vi "Part A.vi"() -> ()   [LabVIEW 2020]
uses:
  <vilib>/MakerHub/LINX/Public/Peripherals/Digital/Digital Write N Chans.vi
  <vilib>/MakerHub/LINX/Private/Local IO/LinxDigitalWrite.vi
  <vilib>/MakerHub/LINX/Public/Utilities/Check Channel.vi
  <vilib>/MakerHub/LINX/Public/Utilities/Open Serial.vi
  <vilib>/MakerHub/LINX/Private/Utilties/Generate Error.vi
  <vilib>/MakerHub/LINX/LMH-LINX.lvlib
panel:
  in  "?":bool
  in  "Serial Port":refnum<visa-resource-name>="N/A"
  in  "Slide":dbl(slide) scale=0.0..4.0
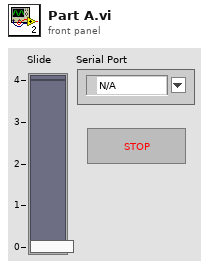
[diagram p1: front panel]
types:
  T1 = typedef "LMH-LINX.lvlib/LINX Ref.ctl" = cluster{"IO":T2, "Interface":T3, "LINX Device Config":T4}
  T2 = typedef "LMH-LINX.lvlib/Platform.ctl" = enum16{"Remote", "Local"}
  T3 = typedef "LMH-LINX.lvlib/Interface.ctl" = enum16{"Serial", "TCP"}
  T4 = typedef "LMH-LINX.lvlib/Device.lvlib/LINX Device Config.ctl" = cluster{"Interface":T3, "COM Port":refnum<visa-resource-name>, "TCP Configuration":T5, "Device Family":u8, "Device ID":u8, "Device Name":string, "TCP Ref":refnum<k5>, "Channels":T6}
  T5 = typedef "LMH-LINX.lvlib/Device.lvlib/TCP Config.ctl" = cluster{"IP Address":string, "Port":u16}
  T6 = typedef "LMH-LINX.lvlib/Channels.ctl" = cluster{"DI":u8[], "DO":u8[], "AI":u8[], "AO":u8[], "PWM":u8[], "QE":u8[], "UART":u8[], "I2C 2":u8[], "SPI":u8[], "CAN":u8[], "Servo":u8[], "AI Ref (V)":dbl, "AI Resolution (Bits)":u8, "AO Ref (V)":dbl, "AO Resolution (Bits)":u8}
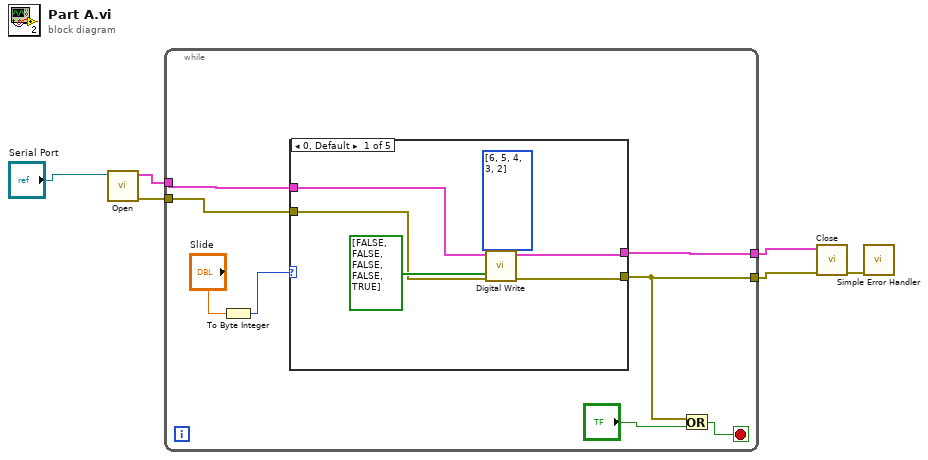
[diagram p0: block diagram]
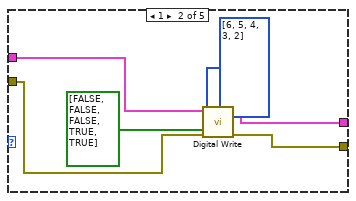
[diagram p2: hidden frame]
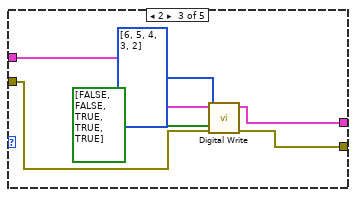
[diagram p3: hidden frame]
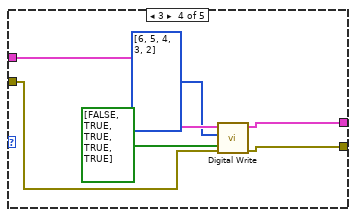
[diagram p4: hidden frame]
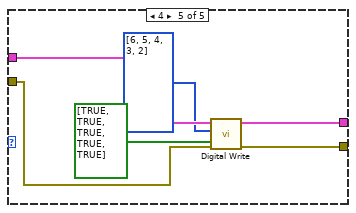
[diagram p5: hidden frame]
diagram:
  n1 = call-poly <vilib>:"Open.vi"("Serial Port"="Serial Port") -> ("Error Out"=w2:errorcluster, "LINX Resource"=w1:T1)  [unwired: 8 in, 1 out]
  n2 = while {
    tunnel: [w12] -> w5
    tunnel: [w14] -> w6
    tunnel: w2 -> [w10]
    tunnel: w1 -> [w9]
    stop <- w13 stop-if-true
    n3 = To Byte Integer(number="Slide") -> (8bit integer=w7:i8)
    n4 = case shown="0, Default" w7 {
      tunnel: w9 -> [w19 w26 w31 w37 w43]
      tunnel: w10 -> [w18 w25 w30 w36 w42]
      tunnel: [w17 w24 w29 w35 w41] -> w14
      tunnel: [w16 w23 w28 w34 w40] -> w12
      frame 0, Default {
        n5 = call-poly <vilib>:"Digital Write.vi"("Error In"=w18, "Values"=bool[] [FALSE, FALSE, FALSE, FALSE, TRUE], "DO Channels"=u8[] [6, 5, 4, 3, 2], "LINX Resource"=w19) -> ("Error Out"=w16:errorcluster, "LINX Resource"=w17:T1)  [unwired: 6 in]
      }
      frame 1 {
        n6 = call-poly <vilib>:"Digital Write.vi"("Error In"=w25, "Values"=bool[] [FALSE, FALSE, FALSE, TRUE, TRUE], "DO Channels"=u8[] [6, 5, 4, 3, 2], "LINX Resource"=w26) -> ("Error Out"=w23:errorcluster, "LINX Resource"=w24:T1)  [unwired: 6 in]
      }
      frame 2 {
        n7 = call-poly <vilib>:"Digital Write.vi"("Error In"=w30, "Values"=bool[] [FALSE, FALSE, TRUE, TRUE, TRUE], "DO Channels"=u8[] [6, 5, 4, 3, 2], "LINX Resource"=w31) -> ("Error Out"=w28:errorcluster, "LINX Resource"=w29:T1)  [unwired: 6 in]
      }
      frame 3 {
        n8 = call-poly <vilib>:"Digital Write.vi"("Error In"=w36, "Values"=bool[] [FALSE, TRUE, TRUE, TRUE, TRUE], "DO Channels"=u8[] [6, 5, 4, 3, 2], "LINX Resource"=w37) -> ("Error Out"=w34:errorcluster, "LINX Resource"=w35:T1)  [unwired: 6 in]
      }
      frame 4 {
        n9 = call-poly <vilib>:"Digital Write.vi"("Error In"=w42, "Values"=bool[] [TRUE, TRUE, TRUE, TRUE, TRUE], "DO Channels"=u8[] [6, 5, 4, 3, 2], "LINX Resource"=w43) -> ("Error Out"=w40:errorcluster, "LINX Resource"=w41:T1)  [unwired: 6 in]
      }
    }
    n10 = Or(x=w12, y="?") -> (x .or. y?=w13:bool)
  }
  n11 = call <vilib>:"Close.vi"("Error In"=w5, "LINX Resource"=w6) -> ("Error Out"=w4:errorcluster)  [unwired: 9 in]
  n12 = call <vilib>:"Simple Error Handler.vi"("error in (no error)"=w4) -> ()  [unwired: 4 in, 5 out]
